vi "APPA109N - Continious measurement.vi"() -> ()   [LabVIEW 2016]
panel:
  out "Current time, s":dbl format="%.2f"
  out "XY Graph":cluster{dbl[], dbl[]}(graph)
  in  "stop":bool
  out "Units":T1(ring)
  out "Number":dbl
  in  "Multimeter Port":refnum<visa-resource-name>="COM3"
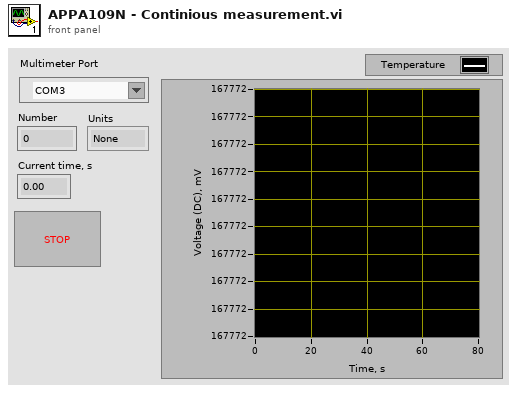
[diagram p1: front panel]
types:
  T1 = enum16{"None", "V", "mV", "A", "mA", "dB", "dBm", "nF", "uF", "mF", "Ohm", "kOhm", "MOhm", "GOhm", "%", "Hz", "kHz", "MHz", "C", "F", "s", "ms", "ns", "V (manual)", "mV (manual)", "A (manual)", "mA (manual)", "Ohm (manual)", "kOhm (maual)", "MOhm (manual)", ""}
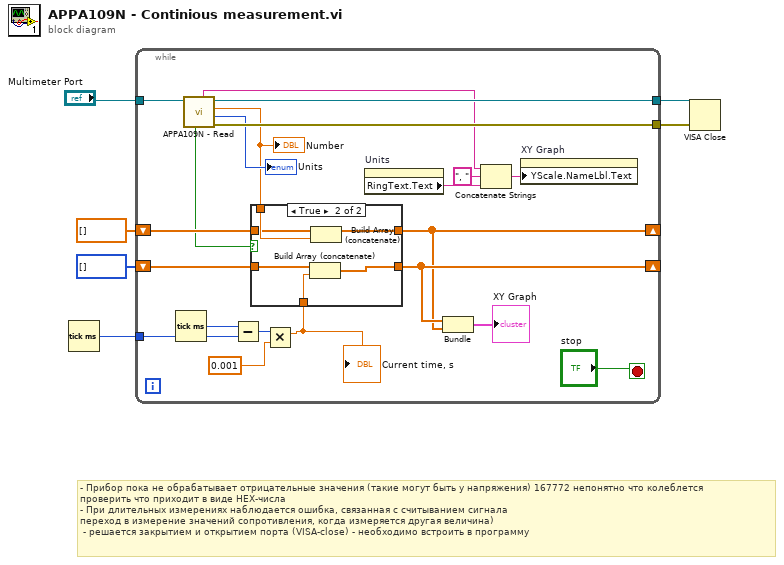
[diagram p0: block diagram]
diagram:
  # "- Прибор пока не обрабатывает отрицательные значения (такие могут быть у напряжения) 167772 непонятно что колеблется\nпроверить что приходит в виде HEX-числа\n- При длительных измерениях наблюдается ошибка, связанная с считыванием сигнала \nпереход в измерение значений сопротивления, когда измеряется другая величина)\n - решается закрытием и открытием порта (VISA-close) - необходимо встроить в программу"
  n1 = Tick Count (ms)() -> (millisecond timer value=w3:u32)
  n2 = while {
    tunnel: "Multimeter Port" -> [w27]
    tunnel: [w26] -> w5
    tunnel: [w25] -> w4
    shift-right: [w17] -> _
    shift-left: dbl[] [] -> [w22]
    tunnel: w3 -> [w14]
    shift-right: [w18] -> _
    shift-left: u32[] [] -> [w19]
    stop <- "stop" stop-if-true
    n3 = Tick Count (ms)() -> (millisecond timer value=w15:u32)
    n4 = call "APPA109N - Read.vi"("VISA resource name"=w27) -> ("error out"=w25:errorcluster, "Units"=→"Units":T1, "Number"=w23:dbl, "VISA resource name out"=w26:refnum<visa-resource-name>, "Regime"=w10:string, "Checksum"=w20:bool)  [unwired: 4 in, 1 out]
    "Number" <- w23
    n5 = Subtract(x=w15, y=w14) -> (x-y=w9:u32)
    n6 = Multiply(x=w9, y=0.001) -> (x*y=w7:dbl)
    "Current time, s" <- w7
    n7 = case shown="True" w20 {
      tunnel: w23 -> [_ w35]
      tunnel: w22 -> [w29 w34]
      tunnel: [w29 w33] -> w17
      tunnel: w19 -> [w28 w32]
      tunnel: w7 -> [_ w31]
      tunnel: [w28 w30] -> w18
      frame False {
      }
      frame True {
        n8 = Build Array (concatenate)(w32, w31) -> (w30:dbl[])
        n9 = Build Array (concatenate)(w34, w35) -> (w33:dbl[])
      }
    }
    n10 = property on="Units" class="Enum (strict)"() -> ("RingText.Text"=w12:string)  [unwired: 2 in, 2 out]
    n11 = Bundle(w18, w17) -> (→"XY Graph":cluster{dbl[], dbl[]})  [unwired: 1 in]
    n12 = Concatenate Strings(w10, ", " ("string"), w12) -> (w13:string)
    n13 = property on="XY Graph" class="XYGraph (strict)"("YScale.NameLbl.Text"=w13) -> ()  [unwired: 2 in, 2 out]
  }
  n14 = VISA Close(VISA resource name=w5, error in (no error)=w4) -> ()  [unwired: 1 out]
